vi "FTW-Test-JSON-Deserialize.vi"() -> (0 "Test Result":errorcluster)   [LabVIEW 2015]
uses:
  src/json/core/FTW-JSON-Core-Type.ctl
  src/reflection/FTW-Reflection-Types.ctl
  src/json/FTW-JSON-Type.ctl
  src/json/core/FTW-JSON-Core-NumericType.vi
  lib/FTW-KernelFilepath.vi
  src/error/FTW-ERR-ThrowError.vi
  src/error/FTW-ERR-ThrowInvalidReferenceError.vi
  src/json/core/FTW-JSON-Core-ElementType.vi
  codegen/xnode/json/fetch/FTW-JSON-Core-GetFlattenedValue.vi
  codegen/xnode/FTW-JSON-Fetch.xnode
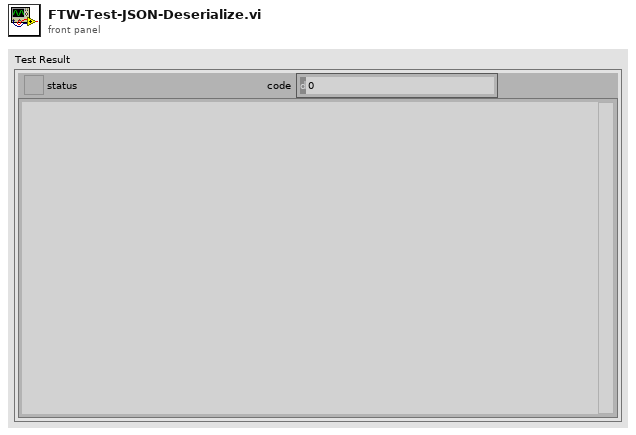
[diagram p1: front panel]
types:
  T1 = typedef "FTW-Type-JSON.ctl" = refnum<data-value>
  T2 = typedef "FTW-JSON-Type.ctl" = enum8{"Not Found", "Object", "Array", "String", "Number", "Boolean", "null"}
  T3 = typedef "FTW-JSON-Core-Type.ctl" = enum8{"Object", "Array", "String", "Integer", "Floating Point", "true", "false", "null", "undefined"}
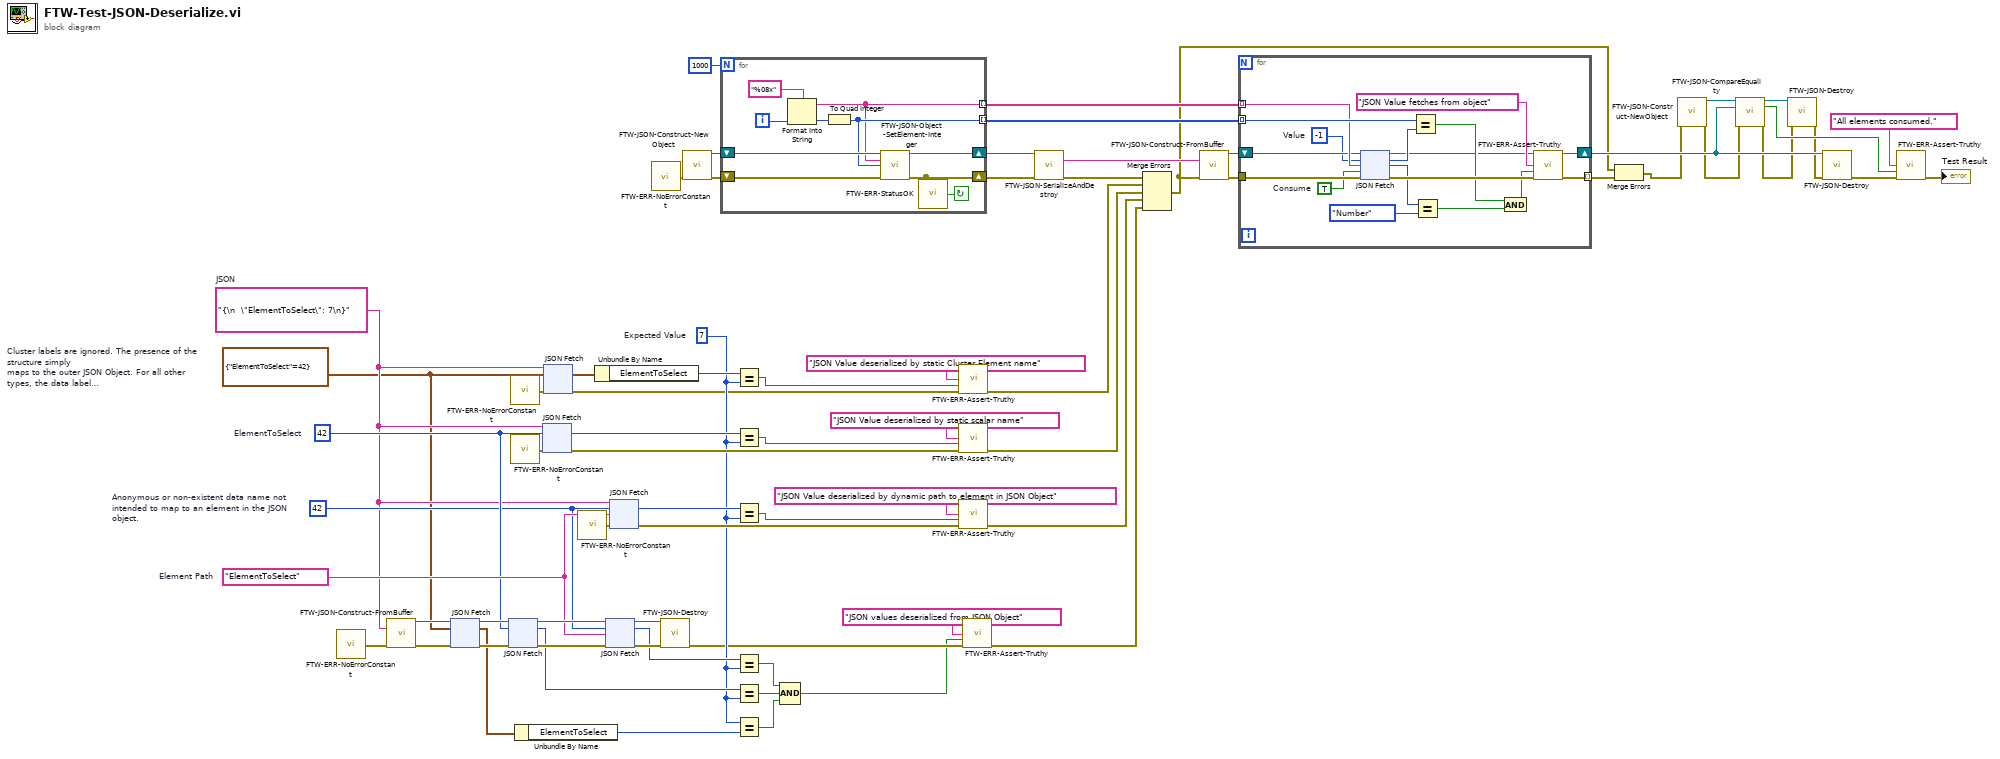
[diagram p0: block diagram]
diagram:
  w7 = 42  # Anonymous or non-existent data name not intended to map to an element in the JSON object.
  w8 = 42  # ElementToSelect
  w21 = "ElementToSelect"  # Element Path
  w35 = 7  # Expected Value
  w4 = "{\n  \"ElementToSelect\": 7\n}"  # JSON
  w3 = cluster{"ElementToSelect":i32} {"ElementToSelect"=42}  # Cluster labels are ignored. The presence of the structure simply maps to the outer JSON Object. For all other types, the data label maps to an element within the implicit outer structure.
  n1 = call "FTW-ERR-NoErrorConstant.vi"() -> ("no error"=w27:errorcluster)
  n2 = call "FTW-JSON-Construct-FromBuffer.vi"("JSON String (UTF-8)"=w4, "error in"=w27) -> ("JSON"=w25:T1, "error out"=w42:errorcluster)  [unwired: 12 in]
  n3 = xnode "JSON Fetch"("JSON"=w25, "Element Type and Default Value"=w3, "error in"=w42) -> ("JSON out"=w24:T1, "Value"=w34:cluster{"ElementToSelect":i32}, "error out"=w39:errorcluster)  [unwired: 2 in, 2 out]
  n4 = xnode "JSON Fetch"("JSON"=w24, "Element Type and Default Value"=w8, "error in"=w39) -> ("JSON out"=w23:T1, "Value"=w37:i32, "error out"=w40:errorcluster)  [unwired: 2 in, 2 out]
  n5 = call "FTW-ERR-NoErrorConstant.vi"() -> ("no error"=w5:errorcluster)
  n6 = call "FTW-ERR-NoErrorConstant.vi"() -> ("no error"=w55:errorcluster)
  n7 = Unbundle By Name(w34) -> ("ElementToSelect"=w33:i32)
  n8 = xnode "JSON Fetch"("JSON"=w4, "Element Type and Default Value"=w8, "error in"=w55) -> ("Value"=w44:i32, "error out"=w49:errorcluster)  [unwired: 2 in, 3 out]
  n9 = xnode "JSON Fetch"("JSON"=w4, "Element Type and Default Value"=w3, "error in"=w5) -> ("Value"=w6:cluster{"ElementToSelect":i32}, "error out"=w26:errorcluster)  [unwired: 2 in, 3 out]
  n10 = call "FTW-ERR-NoErrorConstant.vi"() -> ("no error"=w53:errorcluster)
  n11 = Unbundle By Name(w6) -> ("ElementToSelect"=w54:i32)
  n12 = xnode "JSON Fetch"("JSON"=w23, "Element Type and Default Value"=w7, "Element Path"=w21, "error in"=w40) -> ("JSON out"=w22:T1, "Value"=w36:i32, "error out"=w41:errorcluster)  [unwired: 1 in, 2 out]
  n13 = xnode "JSON Fetch"("JSON"=w4, "Element Type and Default Value"=w7, "Element Path"=w21, "error in"=w53) -> ("Value"=w43:i32, "error out"=w52:errorcluster)  [unwired: 1 in, 3 out]
  n14 = call "FTW-ERR-NoErrorConstant.vi"() -> ("no error"=w70:errorcluster)
  n15 = call "FTW-JSON-Destroy.vi"("JSON"=w22, "error in"=w41) -> ("error out"=w32:errorcluster)  [unwired: 13 in]
  n16 = call "FTW-JSON-Construct-NewObject.vi"("error in"=w70) -> ("JSON"=w69:T1, "error out"=w68:errorcluster)  [unwired: 13 in]
  n17 = for {
    N: 1000 -> [_]
    shift-right: [w74] -> w66
    shift-left: w68 -> [w77]
    shift-right: [w78] -> w9
    shift-left: w69 -> [w79]
    tunnel: [w72] -> w18 mode=indexing
    tunnel: [w71] -> w19 mode=indexing
    i -> [w76]
    stop <- w73 continue-if-true
    n18 = Format Into String(format string="%08x", w76) -> (resulting string=w71:string)  [unwired: 2 in, 1 out]
    n19 = To Quad Integer(1:w76) -> (0:w72:i64)
    n20 = call "FTW-JSON-Object-SetElement-Integer.vi"("JSON"=w79, "Key"=w71, "Value"=w72, "error in"=w77) -> ("JSON out"=w78:T1, "error out"=w74:errorcluster)  [unwired: 10 in]
    n21 = call "FTW-ERR-StatusOK.vi"("error to check"=w74) -> ("Status OK?"=w73:bool)
  }
  n22 = Equal?(x=w54, y=w35) -> (x = y?=w48:bool)
  n23 = Equal?(x=w44, y=w35) -> (x = y?=w50:bool)
  n24 = Equal?(x=w43, y=w35) -> (x = y?=w51:bool)
  n25 = Equal?(x=w36, y=w35) -> (x = y?=w29:bool)
  n26 = Equal?(x=w37, y=w35) -> (x = y?=w31:bool)
  n27 = Equal?(x=w35, y=w33) -> (x = y?=w30:bool)
  n28 = Compound Arithmetic op=AND(w29, w31, w30) -> (w28:bool)
  n29 = call "FTW-ERR-Assert-Truthy.vi"("Assertion"="JSON Value deserialized by static Cluster Element name", "Assertion holds true?"=w48, "error in"=w26) -> ("error out"=w63:errorcluster)  [unwired: 12 in]
  n30 = call "FTW-ERR-Assert-Truthy.vi"("Assertion"="JSON Value deserialized by static scalar name", "Assertion holds true?"=w50, "error in"=w49) -> ("error out"=w64:errorcluster)  [unwired: 12 in]
  n31 = call "FTW-ERR-Assert-Truthy.vi"("Assertion"="JSON Value deserialized by dynamic path to element in JSON Object", "Assertion holds true?"=w51, "error in"=w52) -> ("error out"=w65:errorcluster)  [unwired: 12 in]
  n32 = call "FTW-ERR-Assert-Truthy.vi"("Assertion"="JSON values deserialized from JSON Object", "Assertion holds true?"=w28, "error in"=w32) -> ("error out"=w62:errorcluster)  [unwired: 12 in]
  n33 = call "FTW-JSON-SerializeAndDestroy.vi"("JSON"=w9, "error in"=w66) -> ("JSON String (UTF-8)"=w20:string, "error out"=w61:errorcluster)  [unwired: 12 in]
  n34 = Merge Errors(w61, w63, w64, w65, w62) -> (w1:errorcluster)
  n35 = call "FTW-JSON-Construct-FromBuffer.vi"("JSON String (UTF-8)"=w20, "error in"=w1) -> ("JSON"=w58:T1, "error out"=w59:errorcluster)  [unwired: 12 in]
  n36 = for {
    tunnel: [w92] -> w60 mode=indexing
    tunnel: w59 -> [w95]
    tunnel: w18 -> [w94] mode=indexing
    shift-right: [w81] -> w57
    shift-left: w58 -> [w82]
    tunnel: w19 -> [w83] mode=indexing
    w85 = TRUE  # Consume
    w80 = i64 -1  # Value
    n37 = xnode "JSON Fetch"("JSON"=w82, "Element Type and Default Value"=w80, "Element Path"=w83, "Consume Element"=w85, "error in"=w95) -> ("JSON out"=w81:T1, "Value"=w84:i64, "JSON Element Type"=w90:T2, "error out"=w93:errorcluster)  [unwired: 1 out]
    n38 = Equal?(x=w94, y=w84) -> (x = y?=w87:bool)
    n39 = Equal?(x=w90, y=FTW-JSON-Type."Number") -> (x = y?=w88:bool)
    n40 = And(x=w87, y=w88) -> (x .and. y?=w86:bool)
    n41 = call "FTW-ERR-Assert-Truthy.vi"("Assertion"="JSON Value fetches from object", "Assertion holds true?"=w86, "error in"=w93) -> ("error out"=w92:errorcluster)  [unwired: 12 in]
  }
  n42 = Merge Errors(w1, w60) -> (w56:errorcluster)
  n43 = call "FTW-JSON-Construct-NewObject.vi"("error in"=w56) -> ("JSON"=w17:T1, "error out"=w16:errorcluster)  [unwired: 13 in]
  n44 = call "FTW-JSON-CompareEquality.vi"("JSON"=w17, "JSON to Compare"=w57, "error in"=w16) -> ("JSON out"=w12:T1, "Equal?"=w13:bool, "error out"=w11:errorcluster)  [unwired: 10 in]
  n45 = call "FTW-JSON-Destroy.vi"("JSON"=w12, "error in"=w11) -> ("error out"=w10:errorcluster)  [unwired: 13 in]
  n46 = call "FTW-JSON-Destroy.vi"("JSON"=w57, "error in"=w10) -> ("error out"=w15:errorcluster)  [unwired: 13 in]
  n47 = call "FTW-ERR-Assert-Truthy.vi"("Assertion"="All elements consumed.", "Assertion holds true?"=w13, "error in"=w15) -> ("error out"=→"Test Result":errorcluster)  [unwired: 12 in]
